vi "ProcessHeader.vi"(11 "Array":bool[][](array[boolean])) -> (1 "Number of Bins":u32, 2 "Counts Per Bin":u32, 3 "rTime":u32, 4 "Channel":u32, 5 "Frame Counter":u32, 6 "Sync":u32, 7 "Profiles Per Hist":u32)   [LabVIEW 2012]
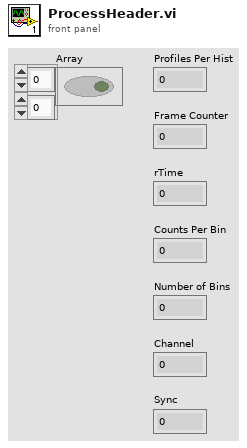
[diagram p1: front panel]
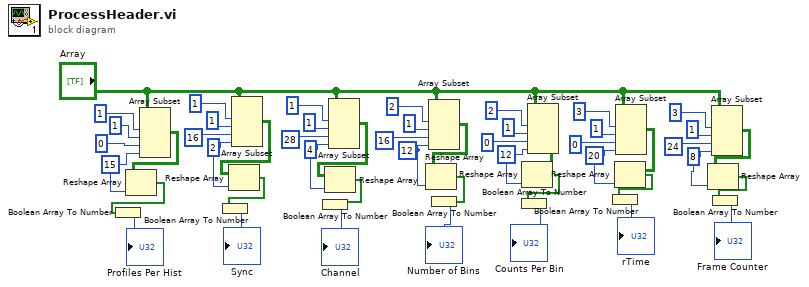
[diagram p0: block diagram]
diagram:
  w39 = 4 ("length")
  w44 = 20 ("length")
  w24 = 12 ("length")
  w20 = 12 ("length")
  w32 = 2 ("length")
  w47 = 8 ("length")
  w28 = 15 ("length")
  n1 = Array Subset(array="Array", index (row)=1 ("index"), length (row)=1 ("length"), index (col)=0 ("index"), length (col)=w28) -> (w27:bool[][])
  n2 = Reshape Array(w27, w28) -> (w25:bool[])
  n3 = Boolean Array To Number(Boolean array=w25) -> (number=→"Profiles Per Hist":u32)
  n4 = Array Subset(array="Array", index (row)=1 ("index"), length (row)=1 ("length"), index (col)=16 ("index"), length (col)=w32) -> (w30:bool[][])
  n5 = Reshape Array(w30, w32) -> (w31:bool[])
  n6 = Boolean Array To Number(Boolean array=w31) -> (number=→"Sync":u32)
  n7 = Array Subset(array="Array", index (row)=1 ("index"), length (row)=1 ("length"), index (col)=28 ("index"), length (col)=w39) -> (w40:bool[][])
  n8 = Reshape Array(w40, w39) -> (w38:bool[])
  n9 = Boolean Array To Number(Boolean array=w38) -> (number=→"Channel":u32)
  n10 = Array Subset(array="Array", index (row)=2 ("index"), length (row)=1 ("length"), index (col)=16 ("index"), length (col)=w20) -> (w19:bool[][])
  n11 = Reshape Array(w19, w20) -> (w49:bool[])
  n12 = Boolean Array To Number(Boolean array=w49) -> (number=→"Number of Bins":u32)
  n13 = Array Subset(array="Array", index (row)=2 ("index"), length (row)=1 ("length"), index (col)=0 ("index"), length (col)=w24) -> (w23:bool[][])
  n14 = Reshape Array(w23, w24) -> (w21:bool[])
  n15 = Boolean Array To Number(Boolean array=w21) -> (number=→"Counts Per Bin":u32)
  n16 = Array Subset(array="Array", index (row)=3 ("index"), length (row)=1 ("length"), index (col)=0 ("index"), length (col)=w44) -> (w43:bool[][])
  n17 = Reshape Array(w43, w44) -> (w41:bool[])
  n18 = Boolean Array To Number(Boolean array=w41) -> (number=→"rTime":u32)
  n19 = Array Subset(array="Array", index (row)=3 ("index"), length (row)=1 ("length"), index (col)=24 ("index"), length (col)=w47) -> (w48:bool[][])
  n20 = Reshape Array(w48, w47) -> (w45:bool[])
  n21 = Boolean Array To Number(Boolean array=w45) -> (number=→"Frame Counter":u32)
